vi "TML-clusters.vi"(7 "RS232-axis":u8=255 format="%0d", 8 "error in (no error)":errorcluster, 9 "value":dbl, 10 "command":string, 11 "axis":u8=255) -> (0 "error out":errorcluster, 1 "expect return":T1(ring), 2 "command byte array":u8[](array[numeric]) format="%02x")   [LabVIEW 2011]
panel:
  in  "Known commands":T2(array[cluster])=[{"command name"="upd", "Parameter"=enum."none", "CommandArray"=[1, 8], "return"=FALSE}, {"command name"="cpa", "Parameter"=enum."none", "CommandArray"=[89, 9, 255, 255, 32, 0], "return"=FALSE}, {"command name"="mode pp3", "Parameter"=enum."none", "CommandArray"=[89, 9, 191, 193, 135, 1], "return"=FALSE}, {"command name"="endinit", "Parameter"=enum."none", "CommandArray"=[0, 32], "return"=FALSE}, {"command name"="axison", "Parameter"=enum."none", "CommandArray"=[1, 2], "return"=FALSE}, {"command name"="axisoff", "Parameter"=enum."none", "CommandArray"=[0, 2], "return"=FALSE}, {"command name"="mode sp", "Parameter"=enum."none", "CommandArray"=[89, 9, 187, 193, 131, 1], "return"=FALSE}, {"command name"="sap", "Parameter"=enum."I32", "CommandArray"=[132, 0], "return"=FALSE}, {"command name"="stop", "Parameter"=enum."none", "CommandArray"=[1, 196], "return"=FALSE}, {"command name"="reset", "Parameter"=enum."none", "CommandArray"=[4, 2], "return"=FALSE}, {"command name"="goto tillcal", "Parameter"=enum."none", "CommandArray"=[116, 0, 64, 11], "return"=FALSE}, {"command name"="goto tillabs", "Parameter"=enum."none", "CommandArray"=[116, 0, 64, 17], "return"=FALSE}, {"command name"="goto tillrange", "Parameter"=enum."none", "CommandArray"=[116, 0, 64, 13], "return"=FALSE}, {"command name"="goto tillstopp", "Parameter"=enum."none", "CommandArray"=[116, 0, 64, 25], "return"=FALSE}, {"command name"="readspi", "Parameter"=enum."I16", "CommandArray"=[176, 8, 0, 17], "return"=TRUE}, {"command name"="writespi@3b0", "Parameter"=enum."I16", "CommandArray"=[144, 168, 3, 176], "return"=FALSE}, {"command name"="goto tillrel", "Parameter"=enum."none", "CommandArray"=[116, 0, 64, 29], "return"=FALSE}, {"command name"="goto @var", "Parameter"=enum."I16", "CommandArray"=[118, 0], "return"=FALSE}, {"command name"="goto bizcal", "Parameter"=enum."none", "CommandArray"=[118, 0, 3, 178], "return"=FALSE}, {"command name"="goto bizrange", "Parameter"=enum."none", "CommandArray"=[118, 0, 3, 179], "return"=FALSE}, {"command name"="goto bizabs", "Parameter"=enum."none", "CommandArray"=[118, 0, 3, 180], "return"=FALSE}, {"command name"="goto bizrel", "Parameter"=enum."none", "CommandArray"=[118, 0, 3, 181], "return"=FALSE}] {"CommandArray" format="%02x"}
  # "format unknown to: @0xFFFF, only 16bit!"
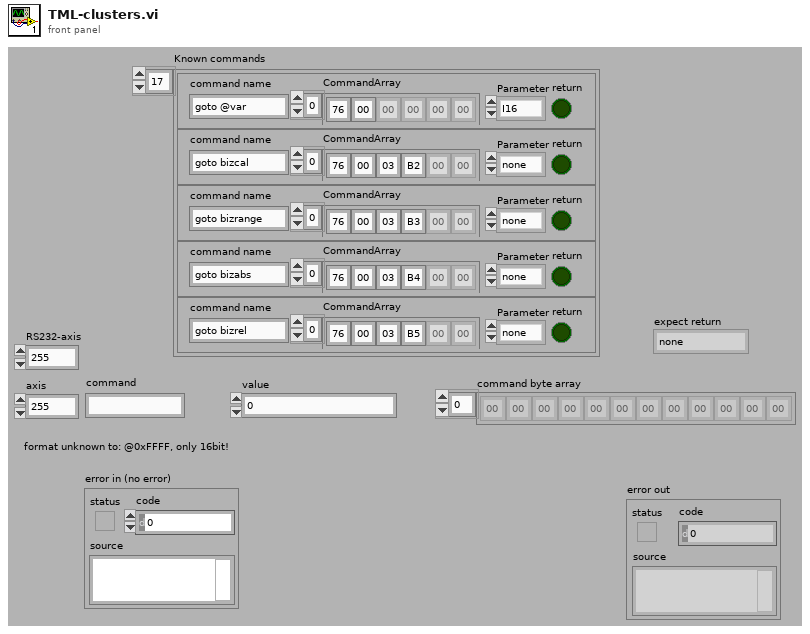
[diagram p1: front panel]
types:
  T1 = enum8{"none", "program", "data", "eprom", "somethingelse"}
  T2 = cluster{"command name":string, "Parameter":enum16{"none", "I16", "I32", "FixedI16.I16", "3Words"}, "CommandArray":u8[], "return":bool}[]
  T3 = enum16{"unknown", "i16", "u16", "i32", "u32", "fix32"}
  T4 = cluster{string[], u32[], enum16{"unknown", "i16", "u16", "i32", "u32", "fix32"}[], "comment":string[]}
  T5 = enum16{"unknown", "i16", "u16", "i32", "u32", "fix32"}[]
  T6 = cluster{"command name":string, "Parameter":enum16{"none", "I16", "I32", "FixedI16.I16", "3Words"}, "CommandArray":u8[], "return":bool}
  T7 = enum16{"none", "I16", "I32", "FixedI16.I16", "3Words"}
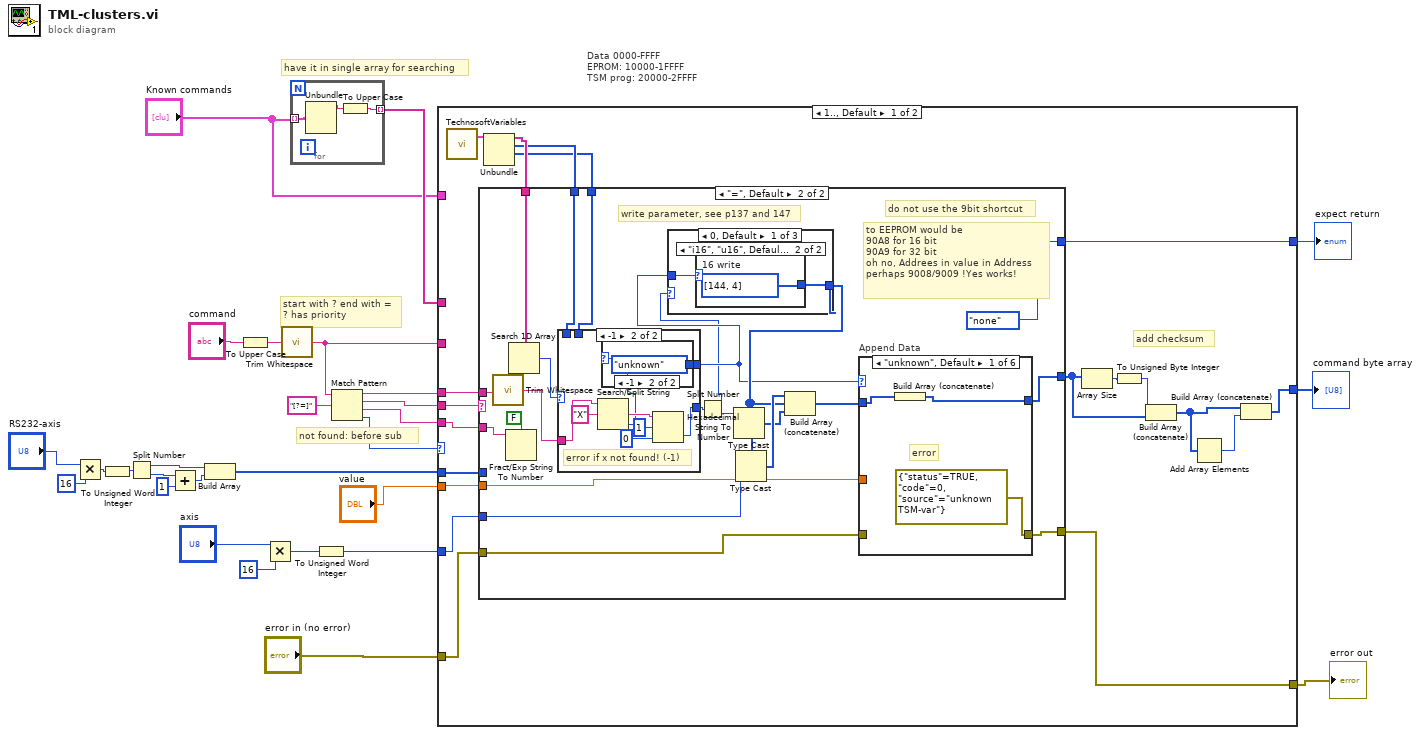
[diagram p0: block diagram]
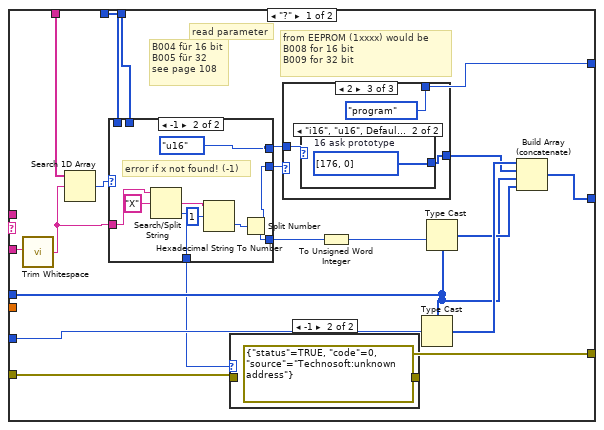
[diagram p2: hidden frame]
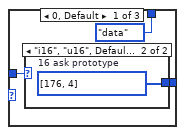
[diagram p4: hidden frame]
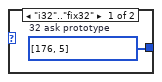
[diagram p5: hidden frame]
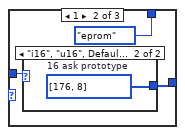
[diagram p6: hidden frame]
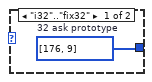
[diagram p7: hidden frame]
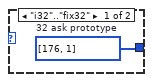
[diagram p8: hidden frame]
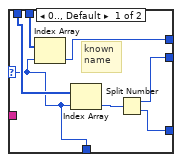
[diagram p9: hidden frame]
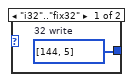
[diagram p10: hidden frame]
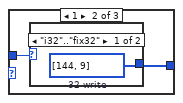
[diagram p11: hidden frame]
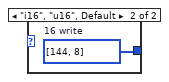
[diagram p12: hidden frame]
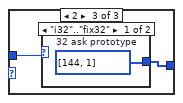
[diagram p13: hidden frame]
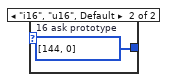
[diagram p14: hidden frame]
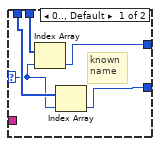
[diagram p15: hidden frame]
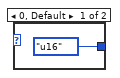
[diagram p16: hidden frame]
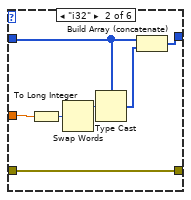
[diagram p17: hidden frame]
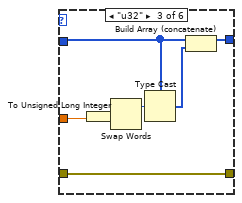
[diagram p18: hidden frame]
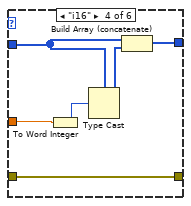
[diagram p19: hidden frame]
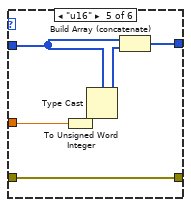
[diagram p20: hidden frame]
diagram:
  # "Data 0000-FFFF\nEPROM: 10000-1FFFF\nTSM prog: 20000-2FFFF"
  # "have it in single array for searching"
  # "not found: before sub"
  # "start with ? end with =\n? has priority"
  n1 = Multiply(x="RS232-axis", y=u16 16) -> (x*y=w13:u16)
  n2 = To Unsigned Word Integer(number=w13) -> (unsigned 16bit integer=w2:u16)
  n3 = Split Number(x=w2) -> (hi(x)=w12:u8, lo(x)=w11:u8)
  n4 = Add(x=w11, y=u8 1) -> (x+y=w10:u8)
  n5 = Build Array(w12, w10) -> (w5:u8[])
  n6 = To Upper Case(1:"command") -> (0:w4:string)
  n7 = Multiply(x="axis", y=u16 16) -> (x*y=w6:u16)
  n8 = call <vilib>:"Trim Whitespace.vi"("string"=w4) -> ("trimmed string"=w24:string)  [unwired: 1 in]
  n9 = for {
    tunnel: "Known commands" -> [w31] mode=indexing
    tunnel: [w29] -> w17 mode=indexing
    n10 = Unbundle(w31) -> ("command name"=w30:string)  [unwired: 3 out]
    n11 = To Upper Case(1:w30) -> (0:w29:string)
  }
  n12 = To Unsigned Word Integer(number=w6) -> (unsigned 16bit integer=w1:u16)
  n13 = Match Pattern(string=w24, regular expression="[?=]") -> (before substring=w21:string, match substring=w20:string, after substring=w19:string, offset past match=w22:i32)  [unwired: 1 out]
  n14 = case shown="1.., Default" w22 {
    tunnel: "error in (no error)" -> [w38 w205]
    tunnel: [w37 w204] -> w26
    tunnel: w24 -> [_ w203]
    tunnel: [w41 w202] -> w23
    tunnel: w21 -> [w49 _]
    tunnel: w20 -> [w50 _]
    tunnel: w19 -> [w48 _]
    tunnel: w1 -> [w47 w201]
    tunnel: "value" -> [w40 w200]
    tunnel: w17 -> [_ w199]
    tunnel: "Known commands" -> [_ w198]
    tunnel: w5 -> [w39 _]
    tunnel: [w32 w197] -> w3
    frame 1.., Default {
      # "add checksum"
      n15 = call "TechnosoftVariables.vi"() -> ("TSM variable table"=w35:T4)  [unwired: 1 in, 3 out]
      n16 = Unbundle(w35) -> (w36:string[], w34:u32[], w33:T5)  [unwired: 1 out]
      n17 = case shown="\"=\", Default" w50 {
        tunnel: w49 -> [_ w119]
        tunnel: w48 -> [w59 w114]
        tunnel: w36 -> [w70 w125]
        tunnel: w34 -> [w69 w111]
        tunnel: w47 -> [w68 w124]
        tunnel: [w64 w120] -> w44
        tunnel: w33 -> [w63 w110]
        tunnel: w40 -> [_ w122]
        tunnel: w39 -> [w60 _]
        tunnel: w38 -> [w52 w118]
        tunnel: [w51 w117] -> w37
        tunnel: [w54 T1."none" ("expect return")] -> w32
        frame "?" {
          # "from EEPROM (1xxxx) would be \nB008 for 16 bit\nB009 for 32 bit"
          # "read parameter"
          # "B004 für 16 bit\nB005 für 32\nsee page 108"
          n18 = call <vilib>:"Trim Whitespace.vi"("string"=w59) -> ("trimmed string"=w57:string)  [unwired: 1 in]
          n19 = Search 1D Array(1D array=w70, element=w57) -> (index of element=w58:i32)  [unwired: 1 out]
          n20 = case shown="-1" w58 {
            selector: w58 -> [w88 _]
            tunnel: w69 -> [w94 _]
            tunnel: [w90 w96] -> w66
            tunnel: w63 -> [w93 _]
            tunnel: [w92 T3."u16" ("type")] -> w62
            tunnel: w57 -> [_ w100]
            tunnel: [w89 w97] -> w55
            tunnel: [w88 w95] -> w53
            frame 0.., Default {
              # "known\nname"
              n21 = Index Array(array=w93, index=w88) -> (element=w92:T3)
              n22 = Index Array(array=w94, index=w88) -> (element=w91:u32)
              n23 = Split Number(x=w91) -> (hi(x)=w89:u16, lo(x)=w90:u16)
            }
            frame -1 {
              # "error if x not found! (-1)"
              n24 = Search/Split String(string=w100, search string/char (-)="X") -> (match + rest of string=w101:string, offset of match=w95:i32)  [unwired: 2 out]
              n25 = Hexadecimal String To Number(string=w101, offset=1) -> (number=w99:u32)  [unwired: 2 out]
              n26 = Split Number(x=w99) -> (hi(x)=w97:u16, lo(x)=w96:u16)
            }
          }
          n27 = case shown="-1" w53 {
            tunnel: w52 -> [w71 _]
            tunnel: [w71 errorcluster {"status"=TRUE, "code"=0, "source"="Technosoft:unknown address"} ("error in (no error)")] -> w51
            frame 0, Default {
            }
            frame -1 {
            }
          }
          n28 = case shown="2" w55 {
            tunnel: w62 -> [w75 w78 w83]
            tunnel: [w74 w80 w84] -> w61
            tunnel: [T1."data" ("expect return") T1."eprom" ("expect return") T1."program" ("expect return")] -> w54
            frame 0, Default {
              n29 = case shown="\"i16\", \"u16\", Default" w75 {
                tunnel: [w76 w77] -> w74
                frame "i32".."fix32" {
                  w76 = u8[] [176, 5]  # 32 ask prototype
                }
                frame "i16", "u16", Default {
                  w77 = u8[] [176, 4]  # 16 ask prototype
                }
              }
            }
            frame 1 {
              n30 = case shown="\"i16\", \"u16\", Default" w78 {
                tunnel: [w81 w82] -> w80
                frame "i32".."fix32" {
                  w81 = u8[] [176, 9]  # 32 ask prototype
                }
                frame "i16", "u16", Default {
                  w82 = u8[] [176, 8]  # 16 ask prototype
                }
              }
            }
            frame 2 {
              n31 = case shown="\"i16\", \"u16\", Default" w83 {
                tunnel: [w86 w87] -> w84
                frame "i32".."fix32" {
                  w86 = u8[] [176, 1]  # 32 ask prototype
                }
                frame "i16", "u16", Default {
                  w87 = u8[] [176, 0]  # 16 ask prototype
                }
              }
            }
          }
          n32 = To Unsigned Word Integer(number=w66) -> (unsigned 16bit integer=w56:u16)
          n33 = Type Cast(type=w60, x=w68) -> (*(type *) &x=w67:u8[])
          n34 = Type Cast(type=w60, x=w56) -> (*(type *) &x=w65:u8[])
          n35 = Build Array (concatenate)(w67, w61, w60, w65) -> (w64:u8[])
        }
        frame "=", Default {
          # "to EEPROM would be \n90A8 for 16 bit\n90A9 for 32 bit\noh no, Addrees in value in Address\nperhaps 9008/9009 !Yes works!"
          # "do not use the 9bit shortcut"
          # "write parameter, see p137 and 147"
          n36 = call <vilib>:"Trim Whitespace.vi"("string"=w119) -> ("trimmed string"=w107:string)  [unwired: 1 in]
          n37 = Fract/Exp String To Number(use system decimal point (T)=FALSE, string=w114) -> ()  [unwired: 4 out]
          n38 = Search 1D Array(1D array=w125, element=w107) -> (index of element=w108:i32)  [unwired: 1 out]
          n39 = case shown="-1" w108 {
            selector: w108 -> [w139 _]
            tunnel: w111 -> [w142 _]
            tunnel: [w138 w143] -> w106
            tunnel: w110 -> [w141 _]
            tunnel: [w140 w146] -> w109
            tunnel: w107 -> [_ w147]
            frame 0.., Default {
              # "known\nname"
              n40 = Index Array(array=w141, index=w139) -> (element=w140:T3)
              n41 = Index Array(array=w142, index=w139) -> (element=w138:u32)
            }
            frame -1 {
              # "error if x not found! (-1)"
              n42 = Search/Split String(string=w147, search string/char (-)="X") -> (match + rest of string=w148:string, offset of match=w144:i32)  [unwired: 2 out]
              n43 = case shown="-1" w144 {
                tunnel: [T3."u16" ("type") T3."unknown" ("type")] -> w146
                frame 0, Default {
                }
                frame -1 {
                }
              }
              n44 = Hexadecimal String To Number(string=w148, offset=1, default (0uL)=u32 0 ("default (0 U32)")) -> (number=w143:u32)  [unwired: 1 out]
            }
          }
          n45 = Split Number(x=w106) -> (hi(x)=w105:u16, lo(x)=w104:u16)
          n46 = case shown="0, Default" w105 {
            tunnel: [w127 w130 w134] -> w115
            tunnel: w109 -> [w126 w131 w135]
            frame 0, Default {
              n47 = case shown="\"i16\", \"u16\", Default" w126 {
                tunnel: [w128 w129] -> w127
                frame "i32".."fix32" {
                  w128 = u8[] [144, 5]  # 32 write
                }
                frame "i16", "u16", Default {
                  w129 = u8[] [144, 4]  # 16 write
                }
              }
            }
            frame 1 {
              n48 = case shown="\"i32\"..\"fix32\"" w131 {
                tunnel: [w132 w133] -> w130
                frame "i32".."fix32" {
                  w132 = u8[] [144, 9]  # 32 write
                }
                frame "i16", "u16", Default {
                  w133 = u8[] [144, 8]  # 16 write
                }
              }
            }
            frame 2 {
              n49 = case shown="\"i32\"..\"fix32\"" w135 {
                tunnel: [w136 w137] -> w134
                frame "i32".."fix32" {
                  w136 = u8[] [144, 1]  # 32 ask prototype
                }
                frame "i16", "u16", Default {
                  w137 = u8[] [144, 0]  # 16 ask prototype
                }
              }
            }
          }
          n50 = Type Cast(type=w115, x=w104) -> (*(type *) &x=w116:u8[])
          n51 = Type Cast(type=w115, x=w124) -> (*(type *) &x=w123:u8[])
          n52 = Build Array (concatenate)(w123, w115, w116) -> (w121:u8[])
          n53 = case "Append Data" shown="\"unknown\", Default" w109 {
            tunnel: w122 -> [_ w162 w169 w171 w177 w195]
            tunnel: w121 -> [w155 w160 w167 w175 w181 w185]
            tunnel: [w154 w159 w166 w173 w179 w196] -> w120
            tunnel: w118 -> [_ w156 w163 w170 w176 w182]
            tunnel: [errorcluster {"status"=TRUE, "code"=0, "source"="unknown TSM-var"} ("error in (no error)") w156 w163 w170 w176 w182] -> w117
            frame "unknown", Default {
              # "error"
              n54 = Build Array (concatenate)(w155) -> (w154:u8[])
            }
            frame "i32" {
              n55 = To Long Integer(number=w162) -> (32bit integer=w157:i32)
              n56 = Swap Words(1:w157) -> (0:w158:i32)
              n57 = Type Cast(type=w160, x=w158) -> (*(type *) &x=w161:u8[])
              n58 = Build Array (concatenate)(w160, w161) -> (w159:u8[])
            }
            frame "u32" {
              n59 = To Unsigned Long Integer(number=w169) -> (unsigned 32bit integer=w164:u32)
              n60 = Swap Words(1:w164) -> (0:w165:u32)
              n61 = Type Cast(type=w167, x=w165) -> (*(type *) &x=w168:u8[])
              n62 = Build Array (concatenate)(w167, w168) -> (w166:u8[])
            }
            frame "i16" {
              n63 = To Word Integer(number=w171) -> (16bit integer=w172:i16)
              n64 = Type Cast(type=w175, x=w172) -> (*(type *) &x=w174:u8[])
              n65 = Build Array (concatenate)(w175, w174) -> (w173:u8[])
            }
            frame "u16" {
              n66 = To Unsigned Word Integer(number=w177) -> (unsigned 16bit integer=w178:u16)
              n67 = Type Cast(type=w181, x=w178) -> (*(type *) &x=w180:u8[])
              n68 = Build Array (concatenate)(w181, w180) -> (w179:u8[])
            }
            frame "fix32" {
              n69 = Quotient & Remainder(x=w195, y=1.0) -> (x-y*floor(x/y)=w187:dbl, floor(x/y)=w193:dbl)
              n70 = Scale By Power Of 2(n=u16 16, x=u32 1) -> (x*2^n=w189:u32)
              n71 = Multiply(x=w189, y=w187) -> (x*y=w188:dbl)
              n72 = To Word Integer(number=w193) -> (16bit integer=w192:i16)
              n73 = To Unsigned Word Integer(number=w188) -> (unsigned 16bit integer=w186:u16)
              n74 = Type Cast(type=w185, x=w186) -> (*(type *) &x=w183:u8[])
              n75 = Type Cast(type=w185, x=w192) -> (*(type *) &x=w184:u8[])
              n76 = Build Array (concatenate)(w185, w183, w184) -> (w196:u8[])
            }
          }
        }
      }
      n77 = Array Size(array=w44) -> (size(s)=w46:i32)
      n78 = To Unsigned Byte Integer(number=w46) -> (unsigned 8bit integer=w45:u8)
      n79 = Build Array (concatenate)(w45, w44) -> (w43:u8[])
      n80 = Add Array Elements(numeric array=w43) -> (sum=w42:u8)
      n81 = Build Array (concatenate)(w43, w42) -> (w41:u8[])
    }
    frame -1 {
      n82 = Search 1D Array(1D array=w199, element=w203) -> (index of element=w206:i32)  [unwired: 1 out]
      n83 = case shown="0.." w206 {
        tunnel: w198 -> [_ w228]
        tunnel: w206 -> [_ w227]
        tunnel: [u8[] [] w218] -> w202
        tunnel: w205 -> [_ w216]
        tunnel: [errorcluster {"status"=TRUE, "code"=0, "source"="unknown TML command"} ("error in (no error)") w216] -> w204
        tunnel: w201 -> [_ w215]
        tunnel: w200 -> [_ w214]
        tunnel: [T1."none" ("expect return") w210] -> w197
        frame -1, Default {
          # "command not found"
        }
        frame 0.. {
          # "expect return seems to be obsolete, always false, only with ?, would need RS232-axis"
          # "•  int    16-bit signed integer \n•  uint   16-bit unsigned integer \n•  fixed  32-bit fixed-point data with the 16MSB for the integer part and the 16LSB \n    for the factionary part.  \n•  long   32-bit signed integer \n•  ulong  32-bit unsigned integer"
          n84 = Index Array(array=w228, index=w227) -> (element=w226:T6)
          n85 = Unbundle(w226) -> ("Parameter"=w217:T7, "CommandArray"=w224:u8[], "return"=w212:bool)  [unwired: 1 out]
          n86 = Type Cast(type=w224, x=w215) -> (*(type *) &x=w225:u8[])
          n87 = case shown="\"none\", Default" w217 {
            tunnel: w225 -> [w231 w238 w244 w259]
            tunnel: w214 -> [_ w237 w239 w257]
            tunnel: w224 -> [w230 w235 w243 w247]
            tunnel: [w229 w234 w241 w258] -> w222
            frame "none", Default {
              n88 = Build Array (concatenate)(w231, w230) -> (w229:u8[])
            }
            frame "I32" {
              n89 = To Long Integer(number=w237) -> (32bit integer=w232:i32)
              n90 = Swap Words(1:w232) -> (0:w233:i32)
              n91 = Type Cast(type=w235, x=w233) -> (*(type *) &x=w236:u8[])
              n92 = Build Array (concatenate)(w238, w235, w236) -> (w234:u8[])
            }
            frame "I16" {
              n93 = To Word Integer(number=w239) -> (16bit integer=w240:i16)
              n94 = Type Cast(type=w243, x=w240) -> (*(type *) &x=w242:u8[])
              n95 = Build Array (concatenate)(w244, w243, w242) -> (w241:u8[])
            }
            frame "FixedI16.I16" {
              n96 = Quotient & Remainder(x=w257, y=1.0) -> (x-y*floor(x/y)=w249:dbl, floor(x/y)=w255:dbl)
              n97 = Scale By Power Of 2(n=u16 16, x=u32 1) -> (x*2^n=w251:u32)
              n98 = Multiply(x=w251, y=w249) -> (x*y=w250:dbl)
              n99 = To Word Integer(number=w255) -> (16bit integer=w254:i16)
              n100 = To Unsigned Word Integer(number=w250) -> (unsigned 16bit integer=w248:u16)
              n101 = Type Cast(type=w247, x=w248) -> (*(type *) &x=w245:u8[])
              n102 = Type Cast(type=w247, x=w254) -> (*(type *) &x=w246:u8[])
              n103 = Build Array (concatenate)(w259, w247, w245, w246) -> (w258:u8[])
            }
          }
          n104 = Array Size(array=w222) -> (size(s)=w223:i32)
          n105 = To Unsigned Byte Integer(number=w223) -> (unsigned 8bit integer=w221:u8)
          n106 = Select(t=T1."somethingelse" ("expect return"), s=w212, f=T1."none" ("expect return")) -> (s? t:f=w210:T1)
          n107 = Build Array (concatenate)(w221, w222) -> (w220:u8[])
          n108 = Add Array Elements(numeric array=w220) -> (sum=w219:u8)
          n109 = Build Array (concatenate)(w220, w219) -> (w218:u8[])
        }
      }
    }
  }
  "error out" <- w26
  "command byte array" <- w23
  "expect return" <- w3
